vi "Folder file.vi"() -> ()   [LabVIEW 2021]
panel:
  out "dup path":path
  out "error out":errorcluster
  out "Path 2":path
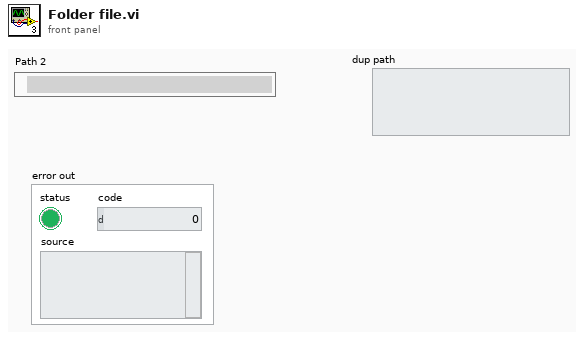
[diagram p1: front panel]
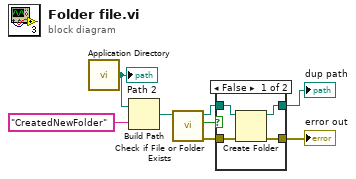
[diagram p0: block diagram]
diagram:
  n1 = call <vilib>:"Application Directory.vi"() -> ("Application Directory"=w8:path)
  "Path 2" <- w8
  n2 = Build Path(base path=w8, name or relative path="CreatedNewFolder") -> (appended path=w7:path)
  n3 = call <vilib>:"Check if File or Folder Exists.vi"("path"=w7) -> ("error out"=w3:errorcluster, "file or folder exists?"=w5:bool, "dup path"=w6:path)  [unwired: 8 in]
  n4 = case shown="False" w5 {
    tunnel: w6 -> [w12 w14]
    tunnel: [w9 w14] -> w1
    tunnel: w3 -> [w11 w13]
    tunnel: [w10 w13] -> w2
    frame False {
      n5 = Create Folder(path (use dialog)=w12, error in=w11) -> (created path=w9:path, error out=w10:errorcluster)  [unwired: 1 in, 1 out]
    }
    frame True {
    }
  }
  "error out" <- w2
  "dup path" <- w1
